vi "LibXML_NavigateAttribute.vi"(8 "error in":errorcluster, 9 "direction":T1, 10 "attribute in":u32) -> (0 "error out":errorcluster, 3 "attribute out":u32)   [LabVIEW 2019, in "Tools.lvlib" / "LibXML.lvlib"]
uses:
  LibXML.lvlib
  LibXML_NavigateDirection.ctl
  dll/lXMLwrap.dll
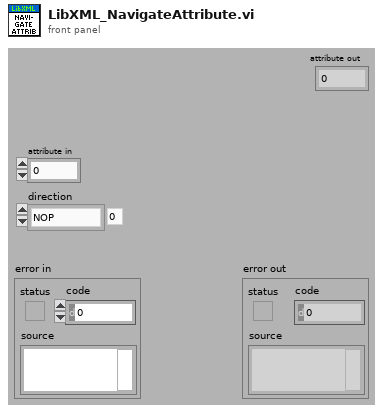
[diagram p1: front panel]
types:
  T1 = typedef "Tools.lvlib/LibXML.lvlib/LibXML_NavigateDirection.ctl" = enum16{"NOP", "first child", "last child", "parent", "next", "prev"}
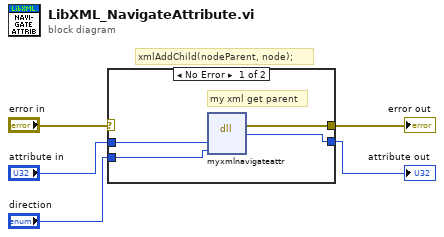
[diagram p0: block diagram]
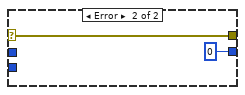
[diagram p2: hidden frame]
diagram:
  # "xmlAddChild(nodeParent, node);"
  n1 = case shown="No Error" "error in" {
    selector: "error in" -> [_ w11]
    tunnel: [w6 w11] -> w4
    tunnel: "attribute in" -> [w9 _]
    tunnel: "direction" -> [w8 _]
    tunnel: [w7 u32 0 ("return type")] -> w1
    frame No Error {
      # "my xml get parent"
      n2 = dll-call lib="C:/Projects/_Prywatne/MyCIT/Framework/Tools/XML/LibXML/dll/lXMLwrap.dll" fn="myxmlnavigateattr"("node"=w9, "type"=w8) -> (error out=w6:errorcluster, "return type"=w7:u32)  [unwired: 5 in, 1 out]
    }
    frame Error {
    }
  }
  "error out" <- w4
  "attribute out" <- w1
